vi "Verify Parameters.vi"(8 "error in (no error)":errorcluster, 10 "night directory":string, 11 "Simulated_CCD_Camera in":refnum<class "Simulated_CCD_Camera.lvclass">) -> (0 "error out":errorcluster, 3 "Simulated_CCD_Camera out":refnum<class "Simulated_CCD_Camera.lvclass">)   [LabVIEW 2018]
uses:
  Simulated_CCD_Camera.lvclass
  Simulated_CCD_Camera.lvclass/Simulated_CCD_Camera.ctl
  <vilib>/CPE Systems NZ Ltd/Error Logger/Error Logger.lvlib
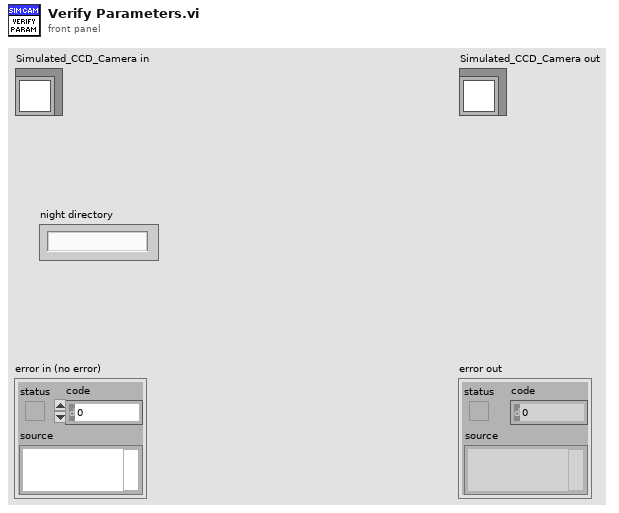
[diagram p1: front panel]
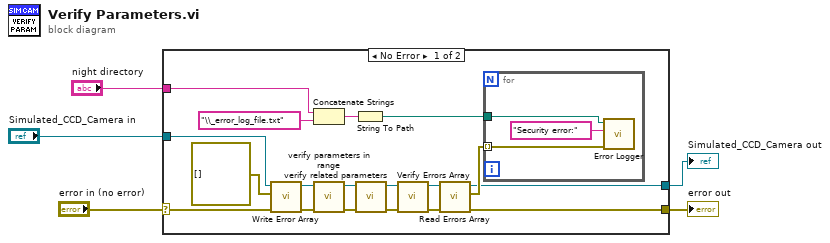
[diagram p0: block diagram]
diagram:
  n1 = case shown="No Error" "error in (no error)" {
    selector: "error in (no error)" -> [w18 w28]
    tunnel: [w8 w28] -> w4
    tunnel: [w9 w27] -> w2
    tunnel: "Simulated_CCD_Camera in" -> [w21 w27]
    tunnel: "night directory" -> [w6 _]
    frame No Error {
      n2 = call "Write Error Array.vi"("error in (no error)"=w18, "Errors array"=errorcluster[] [], "Simulated_CCD_Camera in"=w21) -> ("error out"=w19:errorcluster, "Simulated_CCD_Camera out"=w20:refnum<class "Simulated_CCD_Camera.lvclass">)  [unwired: 7 in]
      n3 = Concatenate Strings(w6, "\\_error_log_file.txt" ("Error Label")) -> (w13:string)
      n4 = call "verify parameters in range.vi"("error in (no error)"=w19, "Simulated_CCD_Camera in"=w20) -> ("error out"=w22:errorcluster, "Simulated_CCD_Camera out"=w23:refnum<class "Simulated_CCD_Camera.lvclass">)  [unwired: 8 in]
      n5 = String To Path(string=w13) -> (path=w7:path)
      n6 = call "verify related parameters.vi"("error in (no error)"=w22, "Simulated_CCD_Camera in"=w23) -> ("error out"=w15:errorcluster, "Simulated_CCD_Camera out"=w16:refnum<class "Simulated_CCD_Camera.lvclass">)  [unwired: 8 in]
      n7 = call "Verify Errors Array.vi"("error in (no error)"=w15, "Simulated_CCD_Camera in"=w16) -> ("error out"=w10:errorcluster, "Simulated_CCD_Camera out"=w11:refnum<class "Simulated_CCD_Camera.lvclass">)  [unwired: 7 in, 1 out]
      n8 = call "Read Errors Array.vi"("error in (no error)"=w10, "Simulated_CCD_Camera in"=w11) -> ("error out"=w8:errorcluster, "Errors array"=w12:errorcluster[], "Simulated_CCD_Camera out"=w9:refnum<class "Simulated_CCD_Camera.lvclass">)  [unwired: 7 in]
      n9 = for {
        tunnel: w12 -> [w25] mode=indexing
        tunnel: w7 -> [w24]
        n10 = call <vilib>:"Error Logger.vi"("Error To Log"=w25, "Error Label"="Security error:", "Custom File Path"=w24) -> ()  [unwired: 7 in, 2 out]
      }
    }
    frame Error {
    }
  }
  "error out" <- w4
  "Simulated_CCD_Camera out" <- w2
